vi "Legend - WaveformChart.vi"(6 "initialize":bool, 8 "error in (no error)":errorcluster, 9 "Plot.Plot Name":string, 10 "Active Plot":i32, 11 "WaveformChart in":refnum<vi>) -> (0 "error out":errorcluster, 1 "Plot.Plot Name":string, 2 "Active Plot":i32, 3 "WaveformChart out":refnum<vi>)   [LabVIEW 2019, in "Instrument.Lockin.lvclass"]
uses:
  Instrument.Lockin.lvclass
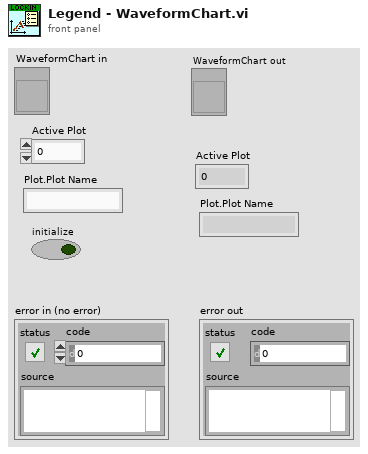
[diagram p1: front panel]
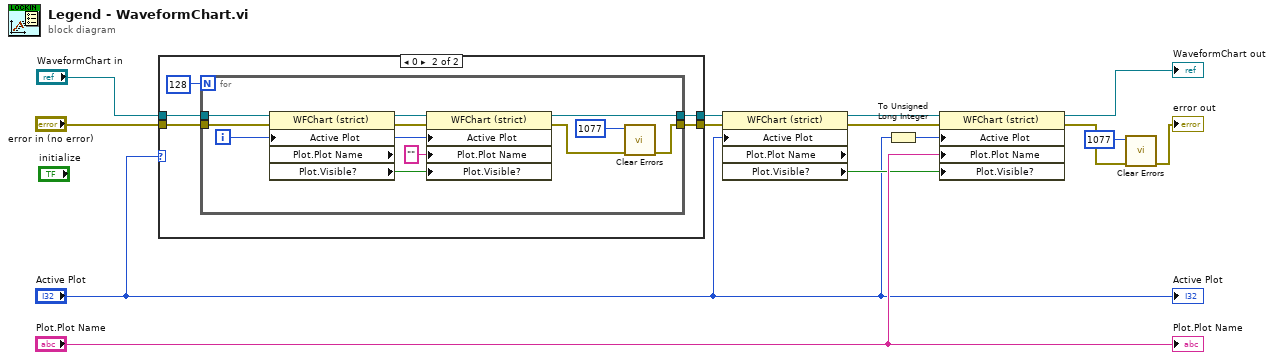
[diagram p0: block diagram]
diagram:
  n1 = case shown="0" "Active Plot" {
    tunnel: "WaveformChart in" -> [w15 w21]
    tunnel: [w16 w20] -> w7
    tunnel: "error in (no error)" -> [w16 w19]
    tunnel: [w15 w17] -> w8
    frame Default {
    }
    frame 0 {
      n2 = for {
        N: 128 -> [_]
        tunnel: w21 -> [w28]
        tunnel: [w31] -> w20
        tunnel: w19 -> [w24]
        tunnel: [w29] -> w17
        i -> [w26]
        n3 = property on="Property Node" class="WFChart (strict)" props=["Active Plot", "Plot", "Plot Name", "Plot", "Visible?"](reference=w28, error in=w24, "Active Plot"=w26) -> (reference out=w27:refnum<vi>, error out=w25:errorcluster, "Plot.Visible?"=w22:bool)  [unwired: 1 out]
        n4 = property on="Property Node" class="WFChart (strict)"(reference=w27, error in=w25, "Active Plot"=w26, "Plot.Plot Name"="" ("format string"), "Plot.Visible?"=w22) -> (reference out=w29:refnum<vi>, error out=w23:errorcluster)
        n5 = call <vilib>:"Clear Errors.vi"("error in (no error)"=w23, "specific error code to clear (0: all)"=1077) -> ("error out"=w31:errorcluster)  [unwired: 4 in, 1 out]
      }
    }
  }
  n6 = property on="Property Node" class="WFChart (strict)" props=["Active Plot", "Plot", "Plot Name", "Plot", "Visible?"](reference=w8, error in=w7, "Active Plot"="Active Plot") -> (reference out=w5:refnum<vi>, error out=w6:errorcluster, "Plot.Visible?"=w4:bool)  [unwired: 1 out]
  n7 = To Unsigned Long Integer(number="Active Plot") -> (unsigned 32bit integer=w10:u32)
  n8 = property on="Property Node" class="WFChart (strict)"(reference=w5, error in=w6, "Active Plot"=w10, "Plot.Plot Name"="Plot.Plot Name", "Plot.Visible?"=w4) -> (reference out=→"WaveformChart out":refnum<vi>, error out=w13:errorcluster)
  n9 = call <vilib>:"Clear Errors.vi"("error in (no error)"=w13, "specific error code to clear (0: all)"=1077) -> ("error out"=→"error out":errorcluster)  [unwired: 4 in, 1 out]
  "Active Plot" <- "Active Plot"
  "Plot.Plot Name" <- "Plot.Plot Name"
